vi "GenerateMatrixPoint.vi"(5 "YOffSet":dbl, 7 "XOffSet":dbl, 8 "error in (no error)":errorcluster, 10 "Pitch":dbl=40.0, 11 "MatrixSize":i32=5) -> (0 "error out":errorcluster, 3 "MatrixPoint":cluster{dbl, dbl}[][](array[cluster]))   [LabVIEW 2019]
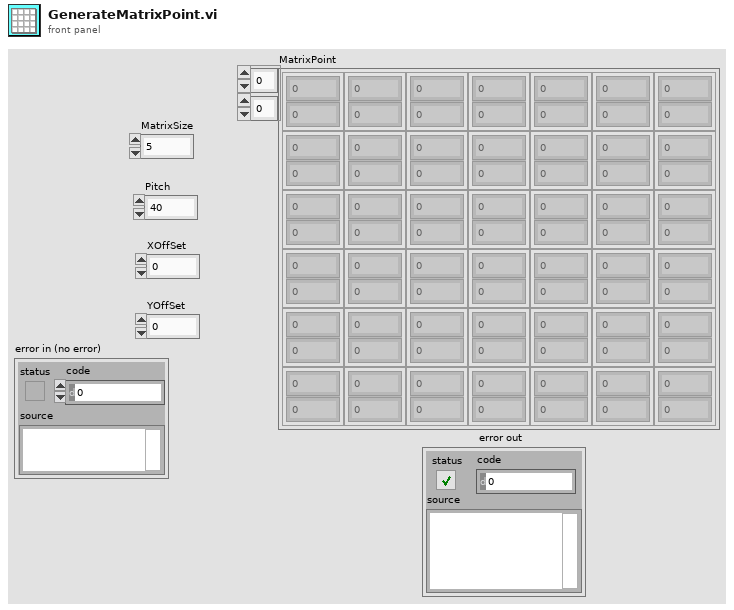
[diagram p1: front panel]
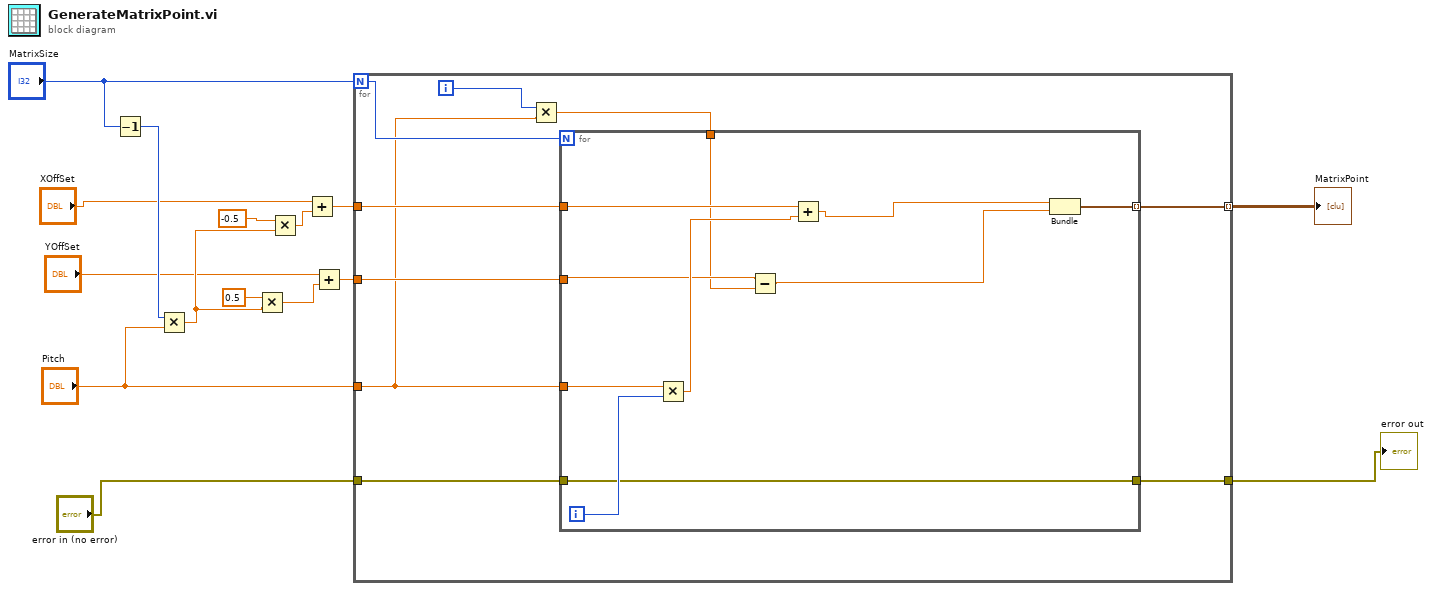
[diagram p0: block diagram]
diagram:
  n1 = Decrement(x="MatrixSize") -> (x-1=w12:i32)
  n2 = Multiply(x=w12, y="Pitch") -> (x*y=w10:dbl)
  n3 = Multiply(x=0.5, y=w10) -> (x*y=w5:dbl)
  n4 = Multiply(x=-0.5, y=w10) -> (x*y=w8:dbl)
  n5 = Add(x="XOffSet", y=w8) -> (x+y=w7:dbl)
  n6 = Add(x="YOffSet", y=w5) -> (x+y=w4:dbl)
  n7 = for {
    N: "MatrixSize" -> [w24]
    tunnel: "Pitch" -> [w18]
    tunnel: w4 -> [w22]
    tunnel: w7 -> [w23]
    tunnel: [w21] -> w15 mode=indexing
    tunnel: [w17] -> w1
    tunnel: "error in (no error)" -> [w16]
    i -> [w20]
    n8 = Multiply(x=w20, y=w18) -> (x*y=w19:dbl)
    n9 = for {
      N: w24 -> [_]
      tunnel: w23 -> [w31]
      tunnel: w22 -> [w28]
      tunnel: [w34] -> w21 mode=indexing
      tunnel: w19 -> [w27]
      tunnel: w18 -> [w32]
      tunnel: [w25] -> w17
      tunnel: w16 -> [w25]
      i -> [w33]
      n10 = Multiply(x=w32, y=w33) -> (x*y=w30:dbl)
      n11 = Subtract(x=w28, y=w27) -> (x-y=w26:dbl)
      n12 = Add(x=w31, y=w30) -> (x+y=w29:dbl)
      n13 = Bundle(w29, w26) -> (w34:cluster{dbl, dbl})  [unwired: 1 in]
    }
  }
  "MatrixPoint" <- w15
  "error out" <- w1
